vi "Close.vi"(8 "error in (no error)":errorcluster, 11 "FLOM Settings in":T1) -> (0 "error out":errorcluster, 3 "FLOM Settings out":T1)   [LabVIEW 2018, in "FLOM Pump.lvlib"]
uses:
  FLOM Pump.lvlib
  Settings Cluster.ctl
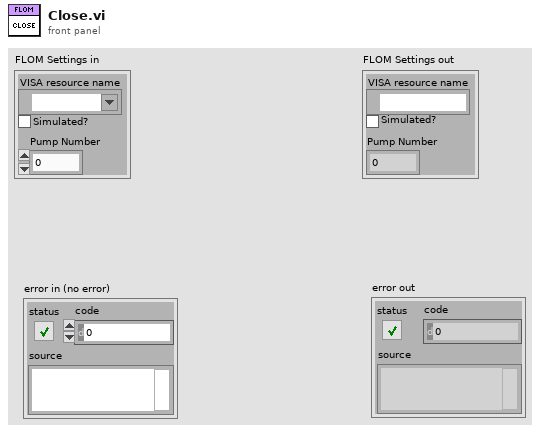
[diagram p1: front panel]
types:
  T1 = typedef "FLOM Pump.lvlib/Settings Cluster.ctl" = cluster{"VISA resource name":refnum<visa-resource-name>, "Simulated?":bool, "Pump Number":dbl}
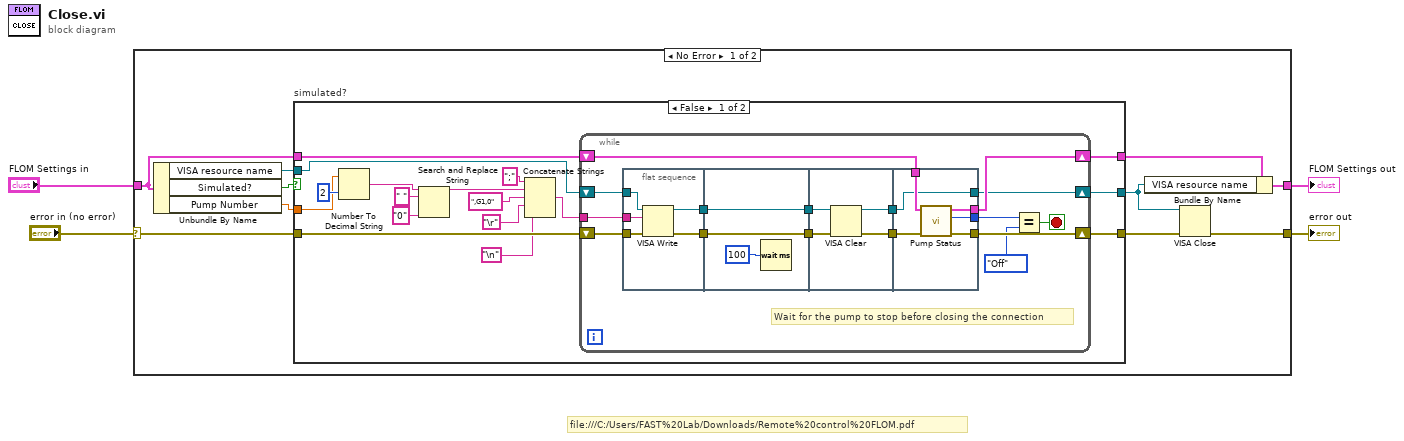
[diagram p0: block diagram]
diagram:
  # "file:///C:/Users/FAST%20Lab/Downloads/Remote%20control%20FLOM.pdf"
  n1 = case shown="No Error" "error in (no error)" {
    selector: "error in (no error)" -> [w11 w70]
    tunnel: [w6 w70] -> w4
    tunnel: [w13 w69] -> w1
    tunnel: "FLOM Settings in" -> [w9 w69]
    frame No Error {
      n2 = Unbundle By Name(w9) -> ("VISA resource name"=w10:refnum<visa-resource-name>, "Simulated?"=w14:bool, "Pump Number"=w12:dbl)
      n3 = case "simulated?" shown="False" w14 {
        tunnel: [w31 w67] -> w7
        tunnel: [w23 w66] -> w5
        tunnel: w12 -> [w16 _]
        tunnel: w11 -> [w27 w67]
        tunnel: w10 -> [w22 w66]
        tunnel: w9 -> [w25 w68]
        tunnel: [w24 w68] -> w8
        frame False {
          n4 = Number To Decimal String(number=w16, width (-)=i16 2) -> (decimal integer string=w19:string)
          n5 = Search and Replace String(input string=w19, search string=" ", replace string="0" ("replace string (\"\")")) -> (result string=w15:string)  [unwired: 5 in, 3 out]
          n6 = Concatenate Strings(";" ("string"), w15, ",G1,0" ("string"), "\r", "\n") -> (w26:string)
          n7 = while {
            tunnel: w26 -> [w40]
            shift-right: [w42] -> w31
            shift-left: w27 -> [w41]
            shift-right: [w38] -> w24
            shift-left: w25 -> [w39]
            shift-right: [w37] -> w23
            shift-left: w22 -> [w35]
            stop <- w33 stop-if-true
            # "Wait for the pump to stop before closing the connection"
            n8 = flat-sequence {
              tunnel: [w48] -> w47
              tunnel: [w49] -> w46
              tunnel: w41 -> [w52]
              tunnel: w40 -> [w51]
              tunnel: w35 -> [w50]
              tunnel: [w55] -> w45
              tunnel: [w54] -> w44
              tunnel: w47 -> [w55]
              tunnel: w46 -> [w54]
              tunnel: w45 -> [w59]
              tunnel: w44 -> [w58]
              tunnel: [w57] -> w43
              tunnel: [w56] -> w36
              tunnel: [w64] -> w42
              tunnel: w43 -> [w65]
              tunnel: w39 -> [w63]
              tunnel: [w62] -> w38
              tunnel: [w61] -> w34
              tunnel: [w60] -> w37
              tunnel: w36 -> [w60]
              frame #0 {
                n9 = VISA Write(VISA resource name=w50, write buffer=w51, error in (no error)=w52) -> (VISA resource name out=w48:refnum<visa-resource-name>, error out=w49:errorcluster)  [unwired: 1 out]
              }
              frame #1 {
                n10 = Wait (ms)(milliseconds to wait=u32 100) -> ()  [unwired: 1 out]
              }
              frame #2 {
                n11 = VISA Clear(VISA resource name=w59, error in (no error)=w58) -> (VISA resource name out=w56:refnum<visa-resource-name>, error out=w57:errorcluster)
              }
              frame #3 {
                n12 = call "Pump Status.vi"("error in (no error)"=w65, "FLOM Settings In"=w63) -> ("error out"=w64:errorcluster, "Pump On?"=w61:enum16{"Off", "On", "Not Initialized"}, "FLOM Settings Out"=w62:T1)  [unwired: 4 in, 3 out]
              }
            }
            n13 = Equal?(x=w34, y=enum16{"Off", "On", "Not Initialized"}."Off") -> (x = y?=w33:bool)
          }
        }
        frame True {
        }
      }
      n14 = Bundle By Name(cluster=w8, "VISA resource name"=w5) -> (w13:T1)
      n15 = VISA Close(VISA resource name=w5, error in (no error)=w7) -> (error out=w6:errorcluster)
    }
    frame Error {
    }
  }
  "error out" <- w4
  "FLOM Settings out" <- w1
